vi "Set Calculation State.vi"(8 "error in (no error)":errorcluster, 10 "Calculation Enabled":bool, 11 "GPU FFT Calculator in":refnum<class "GPU FFT Calculator.lvclass">) -> (0 "error out":errorcluster, 3 "GPU FFT Calculator out":refnum<class "GPU FFT Calculator.lvclass">)   [LabVIEW 2020, in "GPU FFT Calculator.lvlib" / "GPU FFT Calculator.lvclass"]
uses:
  GPU FFT Calculator.lvclass
  Calculation Worker/Calculation Worker/Calculation Worker.lvclass
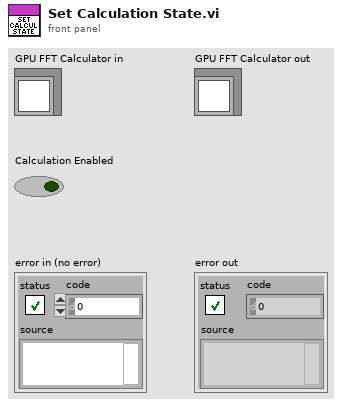
[diagram p1: front panel]
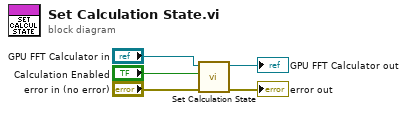
[diagram p0: block diagram]
diagram:
  n1 = call-parent "Set Calculation State.vi"("error in (no error)"="error in (no error)", "Continuous"="Calculation Enabled", "Calculation Worker in"="GPU FFT Calculator in") -> ("error out"=→"error out":errorcluster, "Calculation Worker out"=→"GPU FFT Calculator out":refnum<class "GPU FFT Calculator.lvclass">)  [unwired: 7 in]
